vi "upload_image_sql.vi"() -> ()   [LabVIEW 2022 SP3]
panel:
  out "?":T1(plugin-control)
  in  "Image Path":path
  out "result":string
  out "upload time":string
  out "file size (KB)":dbl
  in  "?":bool
  in  "?":bool
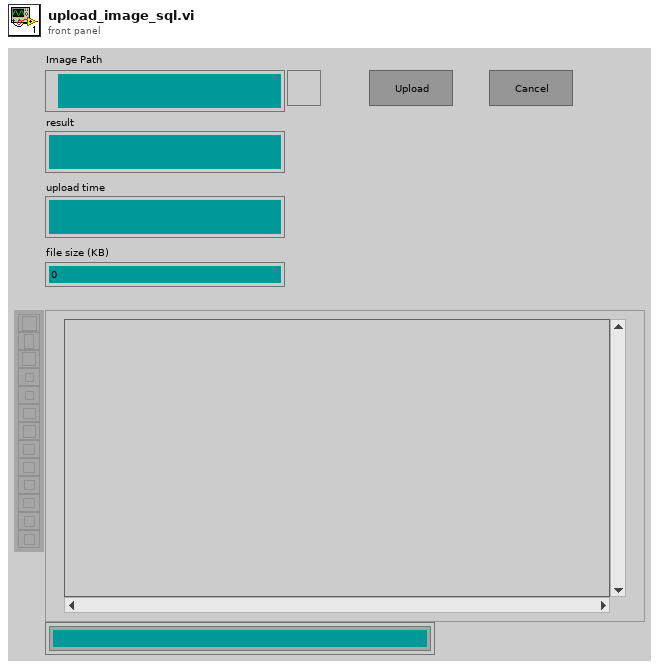
[diagram p1: front panel]
types:
  T1 = typedef "IMAQ Image.ctl" = refnum<image>
  T2 = typedef "Image Type" = u32
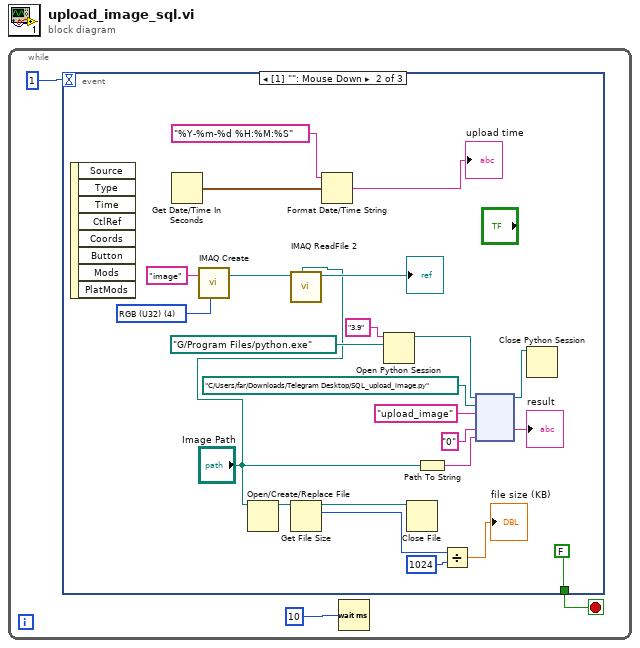
[diagram p0: block diagram]
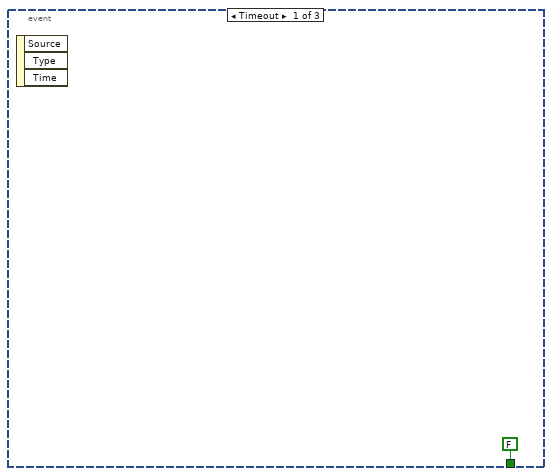
[diagram p2: hidden frame]
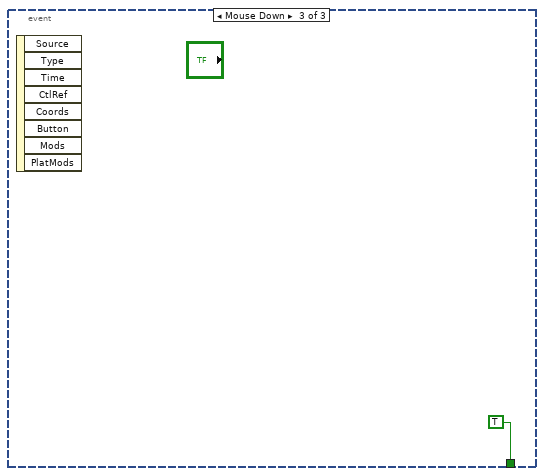
[diagram p3: hidden frame]
diagram:
  n1 = while {
    stop <- w2 stop-if-true
    n2 = event shown="[1] \"\": Mouse Down" {
      selector: _ -> [_ _ _]
      dyn-events: _ -> [_ _ _]
      timeout: 1 -> [_ _ _]
      tunnel: [FALSE FALSE TRUE] -> w2
      event Timeout {
        n3 = event-data() -> ()  [unwired: 1 in, 3 out]
      }
      event Mouse Down {
        w6 = T2 4 items=["Grayscale (U8)", "Grayscale (I16)", "Grayscale (SGL)", "Complex (CSG)", "RGB (U32)", "HSL (U32)", "RGB (U64)", "Grayscale (U16)"] ("Image Type")
        n4 = event-data() -> ()  [unwired: 1 in, 8 out]
        n5 = Get Date/Time In Seconds() -> (seconds since 1Jan1904=w12:timestamp)
        n6 = call "IMAQ Create"("Image Name"="image", "Image Type"=w6) -> ("New Image"=w9:T1)  [unwired: 3 in, 1 out]
        n7 = Open/Create/Replace File(file path (use dialog)="Image Path") -> (refnum out=w24:refnum<file>)  [unwired: 5 in, 2 out]
        n8 = call "IMAQ ReadFile 2"("File Path"="Image Path", "Image"=w9) -> ("Image Out"=→"?":T1)  [unwired: 5 in, 4 out]
        n9 = Get File Size(file=w24) -> (refnum out=w13:refnum<file>, size (in bytes)=w27:i64)  [unwired: 1 in, 1 out]
        n10 = Format Date/Time String(time format string (%c)="%Y-%m-%d %H:%M:%S", seconds (now)=w12) -> (date/time string=→"upload time":string)  [unwired: 1 in]
        n11 = Open Python Session(python version="3.9" ("Python version"), python path=path "G:/Program Files/python.exe" ("Python path")) -> (session out=w19:refnum<k35>)  [unwired: 1 in, 1 out]
        n12 = Close File(refnum=w13) -> ()  [unwired: 1 in, 2 out]
        n13 = Path To String(path="Image Path") -> (string=w16:string)
        n14 = Divide(x=w27, y=i64 1024) -> (x/y=→"file size (KB)":dbl)
        n15 = node(w19, path "C:/Users/far/Downloads/Telegram Desktop/SQL_upload_image.py" ("module path"), "upload_image" ("function name"), "0", w16) -> (w18:refnum<k35>, →"result":string)  [unwired: 2 in, 3 out]
        n16 = Close Python Session(session in=w18) -> ()  [unwired: 1 in, 1 out]
      }
      event Mouse Down {
        n17 = event-data() -> ()  [unwired: 1 in, 8 out]
      }
    }
    n18 = Wait (ms)(milliseconds to wait=u32 10) -> ()  [unwired: 1 out]
  }
